vi "standard request and response.vi"(6 "source if error":string, 7 "ignore response":bool, 8 "error in":errorcluster, 9 "timeout (-1)":i32=-1, 10 "request":T3, 11 "Standard Engine Runtime in":refnum<class "Standard Engine Runtime.lvclass">) -> (0 "error out":errorcluster, 2 "message from engine":T1, 3 "Standard Engine Runtime out":refnum<class "Standard Engine Runtime.lvclass">)   [LabVIEW 2013, in "Standard Engine Runtime.lvclass"]
uses:
  Standard Engine Runtime.lvclass
  main engine/message to engine.ctl
  main engine/message request type.ctl
  main engine/message from engine.ctl
  main engine/message response type.ctl
  Standard Engine Runtime.lvclass/Standard Engine Runtime.ctl
  main engine/main engine.lvlib
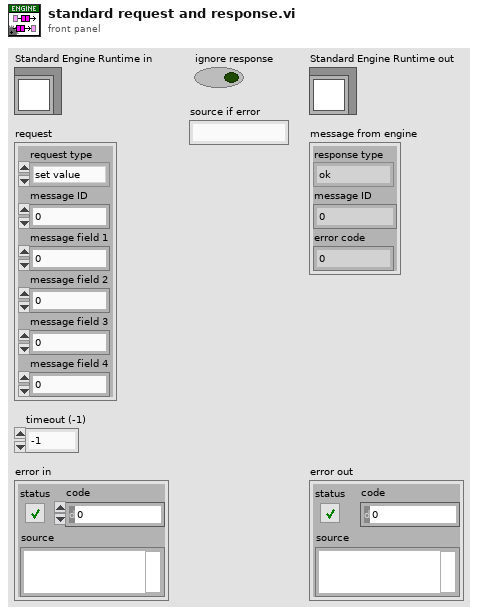
[diagram p1: front panel]
types:
  T1 = typedef "main engine.lvlib/message from engine.ctl" = cluster{"response type":T2, "message ID":u8, "error code":i32}
  T2 = typedef "main engine.lvlib/message response type.ctl" = enum8{"ok", "error"}
  T3 = typedef "main engine.lvlib/message to engine.ctl" = cluster{"request type":T4, "message ID":u8, "message field 1":u64, "message field 2":u64, "message field 3":u64, "message field 4":u64}
  T4 = typedef "main engine.lvlib/message request type.ctl" = enum8{"set value", "disable module", "enable module"}
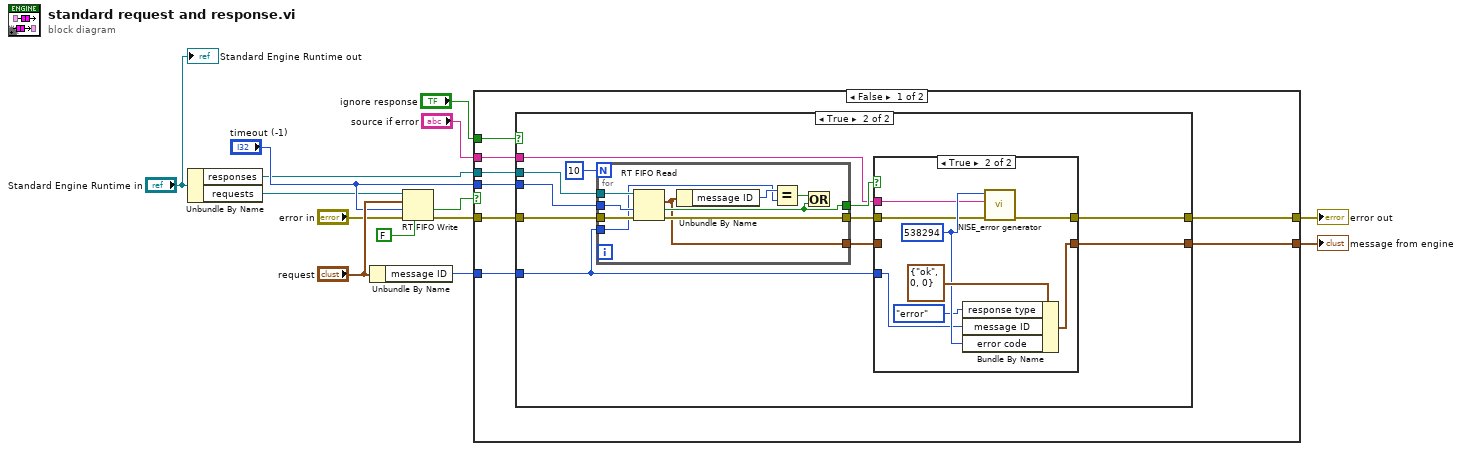
[diagram p0: block diagram]
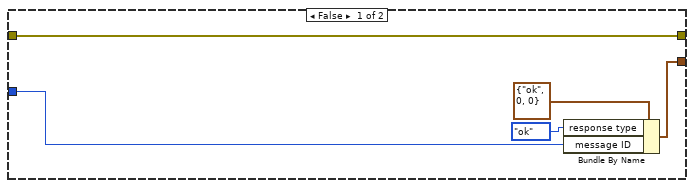
[diagram p2: hidden frame]
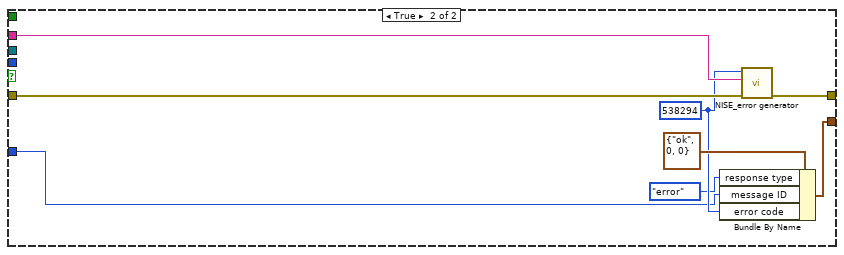
[diagram p4: hidden frame]
diagram:
  n1 = Unbundle By Name("Standard Engine Runtime in") -> ("responses"=w6:refnum<k33>, "requests"=w5:refnum<k33>)
  n2 = Unbundle By Name("request") -> ("message ID"=w14:u8)
  n3 = RT FIFO Write(0:w5, 1:"request", 2:"timeout (-1)", 3:"error in", 5:FALSE ("overwrite on timeout (T)")) -> (10:w9:bool, 11:w3:errorcluster)  [unwired: 2 out]
  n4 = case shown="False" w9 {
    tunnel: w3 -> [w22 w65]
    tunnel: [w21 w64] -> w4
    tunnel: w6 -> [w20 _]
    tunnel: "timeout (-1)" -> [w19 _]
    tunnel: "source if error" -> [w15 w63]
    tunnel: "ignore response" -> [w18 _]
    tunnel: [w17 w61] -> w12
    tunnel: w14 -> [w16 w59]
    frame False {
      n5 = case shown="True" w18 {
        tunnel: w22 -> [w27 w38]
        tunnel: [w27 w34] -> w21
        tunnel: w20 -> [_ w37]
        tunnel: w19 -> [_ w36]
        tunnel: [w25 w31] -> w17
        tunnel: w16 -> [w24 w29]
        tunnel: w15 -> [_ w30]
        frame False {
          n6 = Bundle By Name(cluster=T1 {"response type"=enum."ok", "message ID"=0, "error code"=0} ("message from engine"), "response type"=message_response_type."ok", "message ID"=w24) -> (w25:T1)
        }
        frame True {
          n7 = for {
            N: 10 -> [_]
            tunnel: w38 -> [w47]
            tunnel: w37 -> [w46]
            tunnel: w36 -> [w45]
            tunnel: [w43] -> w35
            tunnel: [w44] -> w33
            tunnel: [w41] -> w32
            tunnel: w29 -> [w39]
            n8 = RT FIFO Read(0:w46, 2:w45, 3:w47) -> (9:w41:T1, 10:w43:bool, 11:w44:errorcluster)  [unwired: 1 in, 2 out]
            n9 = Unbundle By Name(w41) -> ("message ID"=w40:u8)
            n10 = Equal?(x=w40, y=w39) -> (x = y?=w42:bool)
            n11 = Or(x=w42, y=w43) -> ()  [unwired: 1 out]
          }
          n12 = case shown="True" w35 {
            tunnel: [w49 w53] -> w34
            tunnel: w33 -> [w49 w54]
            tunnel: w32 -> [w48 _]
            tunnel: [w48 w52] -> w31
            tunnel: w29 -> [_ w51]
            tunnel: w30 -> [_ w50]
            frame False {
            }
            frame True {
              w56 = 538294 ("error code (0)")
              n13 = Bundle By Name(cluster=T1 {"response type"=enum."ok", "message ID"=0, "error code"=0} ("message from engine"), "response type"=message_response_type."error", "message ID"=w51, "error code"=w56) -> (w52:T1)
              n14 = call <vilib>:"NISE_error generator.vi"("error in"=w54, "append error message"=w50, "error code (0)"=w56) -> ("error out"=w53:errorcluster)  [unwired: 6 in]
            }
          }
        }
      }
    }
    frame True {
      w60 = 538294 ("error code (0)")
      n15 = Bundle By Name(cluster=T1 {"response type"=enum."ok", "message ID"=0, "error code"=0} ("message from engine"), "response type"=message_response_type."error", "message ID"=w59, "error code"=w60) -> (w61:T1)
      n16 = call <vilib>:"NISE_error generator.vi"("error in"=w65, "append error message"=w63, "error code (0)"=w60) -> ("error out"=w64:errorcluster)  [unwired: 6 in]
    }
  }
  "message from engine" <- w12
  "error out" <- w4
  "Standard Engine Runtime out" <- "Standard Engine Runtime in"
